vi "FPGA_target_command_handler.vi"(0 "mem_addr_in":u32, 1 "mem_addr_start":u32, 3 "force_stop":bool, 4 "stop_execution_in":bool, 5 "FIFO_full":bool, 6 "continuous":bool, 7 "mem_data_in":T1) -> (10 "mem2_addr":u32, 11 "start_sctl":bool, 12 "mem2_data":u16, 13 "mem_data_out":T1, 14 "mem_addr_ out":u32, 17 "stop_execution_out":bool, 18 "stop_triggered":bool, 19 "write_FIFO":bool)   [LabVIEW 2014]
doc: "Reads data from the internal memory of the FPGA and provides output that will be used later-on to be filled into an internal FIFO"
uses:
  FPGA_mem_data_type.ctl
panel:
  # "<-- renamed"
  # "<-- renamed"
  # "--> new control/ indicator which are connected to new shift-register <--"
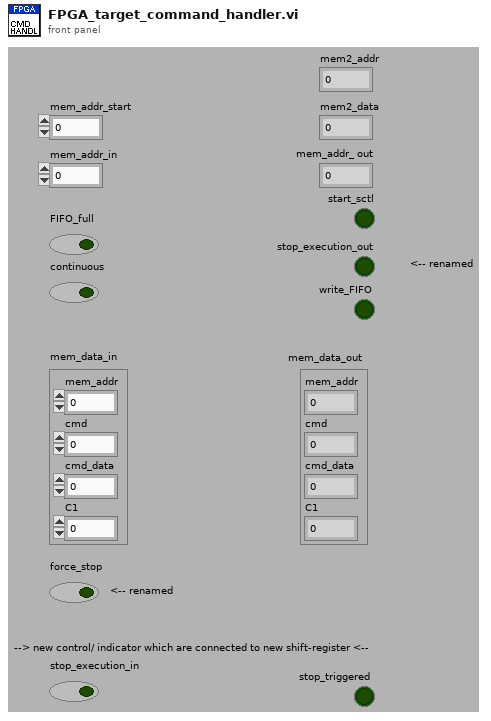
[diagram p1: front panel]
types:
  T1 = typedef "FPGA_mem_data_type.ctl" = cluster{"mem_addr":u32, "cmd":u8, "cmd_data":u32, "C1":u16}
  T2 = cluster{"addr_dup":u32, "Mem 0 data":u8, "data_mem3":u32, "data_mem2":u16}
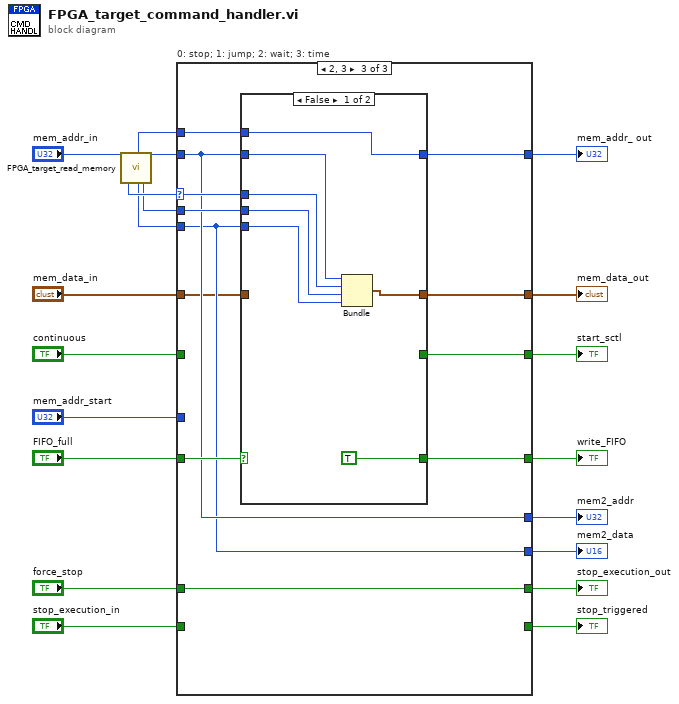
[diagram p0: block diagram]
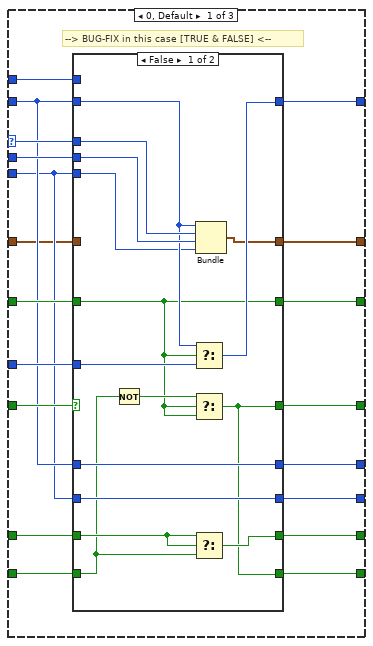
[diagram p2: hidden frame]
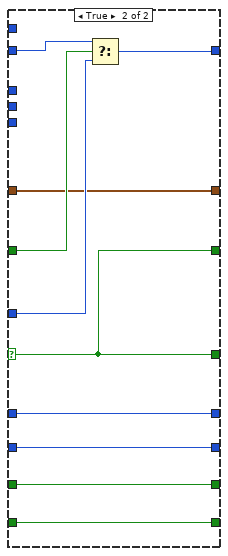
[diagram p3: hidden frame]
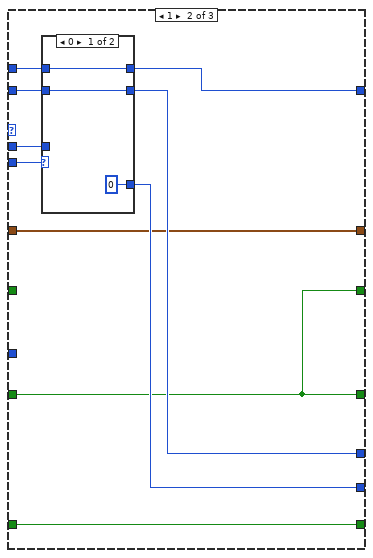
[diagram p4: hidden frame]
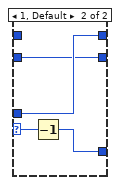
[diagram p5: hidden frame]
diagram:
  n1 = call "FPGA_target_read_memory.vi"("addr_in"="mem_addr_in") -> ("data_mem0"=w12:u8, "next_addr_out"=w8:u32, "data_mem2"=w9:u16, "data_mem3"=w10:u32, "addr_dup"=w11:u32)  [unwired: 14 in]
  n2 = case "0: stop; 1: jump; 2: wait; 3: time" shown="2, 3" w12 {
    selector: w12 -> [w34 _ w90]
    tunnel: w11 -> [w27 w74 w85]
    tunnel: [w38 w70 w87] -> w5
    tunnel: w9 -> [w25 w72 w84]
    tunnel: [w36 w65 w86] -> w20
    tunnel: [w37 w65 w91] -> w18
    tunnel: w10 -> [w33 w73 w89]
    tunnel: "continuous" -> [w32 _ _]
    tunnel: "mem_addr_start" -> [w31 _ _]
    tunnel: "FIFO_full" -> [w39 w65 w92]
    tunnel: w8 -> [w35 w71 w88]
    tunnel: "force_stop" -> [w30 w69 w93]
    tunnel: [w29 w69 w93] -> w13
    tunnel: [w28 w68 w85] -> w7
    tunnel: [w26 w67 w84] -> w6
    tunnel: [w23 w66 w83] -> w4
    tunnel: "mem_data_in" -> [w24 w66 w82]
    tunnel: "stop_execution_in" -> [w22 _ _]
    tunnel: [w21 _ _] -> w1
    frame 0, Default {
      # "--> BUG-FIX in this case [TRUE & FALSE] <--"
      n3 = case shown="False" w39 {
        selector: w39 -> [_ w64]
        tunnel: w27 -> [w49 w57]
        tunnel: [w47 w60] -> w38
        tunnel: [w43 w64] -> w37
        tunnel: [w42 w64] -> w36
        tunnel: w35 -> [_ _]
        tunnel: w34 -> [w51 _]
        tunnel: w33 -> [w50 _]
        tunnel: w25 -> [w41 _]
        tunnel: w32 -> [w42 w59]
        tunnel: w31 -> [w48 w58]
        tunnel: w30 -> [w54 w63]
        tunnel: [w44 w63] -> w29
        tunnel: w27 -> [w53 w62]
        tunnel: [w53 w62] -> w28
        tunnel: w25 -> [w52 w61]
        tunnel: [w52 w61] -> w26
        tunnel: w24 -> [_ w56]
        tunnel: [w40 w56] -> w23
        tunnel: w22 -> [w45 w55]
        tunnel: [w43 w55] -> w21
        frame False {
          n4 = Not(x=w45) -> (.not. x?=w46:bool)
          n5 = Select(t=w49, s=w42, f=w48) -> (s? t:f=w47:u32)
          n6 = Select(t=w46, s=w42, f=w42) -> (s? t:f=w43:bool)
          n7 = Select(t=w54, s=w54, f=w45) -> (s? t:f=w44:bool)
          n8 = Bundle("addr_dup"=w49, "Mem 0 data"=w51, "data_mem3"=w50, "data_mem2"=w41) -> (w40:T2)  [unwired: 1 in]
        }
        frame True {
          n9 = Select(t=w57, s=w59, f=w58) -> (s? t:f=w60:u32)
        }
      }
    }
    frame 1 {
      n10 = case shown="0" w72 {
        selector: w72 -> [_ w80]
        tunnel: [w77 w81] -> w70
        tunnel: w74 -> [w76 w79]
        tunnel: w73 -> [_ w81]
        tunnel: w71 -> [w77 _]
        tunnel: [w76 w79] -> w68
        tunnel: [u16 0 w78] -> w67
        frame 0 {
        }
        frame 1, Default {
          n11 = Decrement(x=w80) -> (x-1=w78:u16)
        }
      }
    }
    frame 2, 3 {
      n12 = case shown="False" w92 {
        selector: w92 -> [_ w103]
        tunnel: [TRUE w103] -> w91
        tunnel: w90 -> [w97 _]
        tunnel: w89 -> [w96 _]
        tunnel: w84 -> [w95 _]
        tunnel: w88 -> [w100 _]
        tunnel: [w100 w102] -> w87
        tunnel: w85 -> [w98 w102]
        tunnel: [_ w103] -> w86
        tunnel: [w94 w101] -> w83
        tunnel: w82 -> [_ w101]
        frame False {
          n13 = Bundle("addr_dup"=w98, "Mem 0 data"=w97, "data_mem3"=w96, "data_mem2"=w95) -> (w94:T2)  [unwired: 1 in]
        }
        frame True {
        }
      }
    }
  }
  "mem_addr_ out" <- w5
  "start_sctl" <- w20
  "write_FIFO" <- w18
  "stop_execution_out" <- w13
  "mem2_addr" <- w7
  "mem2_data" <- w6
  "mem_data_out" <- w4
  "stop_triggered" <- w1
